vi "Arm Control.vi"(8 "error in (no error)":errorcluster) -> ()   [LabVIEW 2013]
uses:
  Robot Global Data.vi
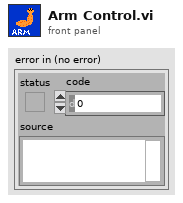
[diagram p1: front panel]
types:
  T1 = typedef "WPI_MotorControlDeviceRef.ctl" = cluster{"DeviceStatus":errorcluster, "Type":enum16{"PWM", "CAN"}, "PWM":cluster{"Digital Module":T2, "PWM Channel":T3, "DeadBand":T4}, "CAN":cluster{"Device Number":u8, "Control Mode":T5, "Semaphore":T6, "Max Vout":dbl}, "Invert":bool, "TransformRef":T7, "InvTransformRef":T7}
  T2 = typedef "FPGA_TypedefDigitalModule.ctl" = enum16{"Digital Module 1", "Digital Module 2"}
  T3 = typedef "FPGA_DIOPWMChannel.ctl" = enum8{"PWM 1", "PWM 2", "PWM 3", "PWM 4", "PWM 5", "PWM 6", "PWM 7", "PWM 8", "PWM 9", "PWM 10", "Invalid"}
  T4 = typedef "WPI_PWMDeadband.ctl" = cluster{"Name":string, "maxPositivePwm":i32, "minPositivePwm":i32, "centerPwm":i32, "maxNegativePwm":i32, "minNegativePwm":i32, "angularRange":u16}
  T5 = typedef "WPI_CANJaguar_ControlMode.ctl" = enum8{"Percent VBus", "Current", "Speed", "Position", "Voltage"}
  T6 = typedef "Semaphore RefNum" = refnum<k1>
  T7 = typedef "WPI_PWMTransform_ConPane.ctl" = refnum<vi>
  T8 = typedef "User Commands typedef.ctl" = cluster{"Arm Command":T9, "Shooter Commands":T11, "Drive Commands":T12}
  T9 = typedef "Arm control typedef.ctl" = cluster{"Arm up/dwn":dbl, "Arm Capture":bool, "Arm Pass":bool, "Arm Positions":T10, "Arm Manual Override":bool}
  T10 = typedef "Arm Postions Enum Typedef.ctl" = enum16{"Arm Pick-up", "Arm Shoot", "Arm Truss", "Manual"}
  T11 = typedef "Shooter Commands Typedef.ctl" = cluster{"Shooter Fire":bool, "Shooter Draw":bool}
  T12 = typedef "Drive Commands Typedef.ctl" = cluster{"Drive L/R":dbl, "Drive Fwd/Rev":dbl}
  T13 = typedef "Robot Info Typedef.ctl" = cluster{"Arm Info":T14, "Shooter Info":T15}
  T14 = typedef "Arm Info Typedef.ctl" = cluster{"Current Arm Position":dbl, "Arm Bottom Limit Switch":bool, "Arm Top Limit Switch":bool}
  T15 = typedef "Shooter Info Typedef.ctl" = cluster{"Shooter At Full":bool}
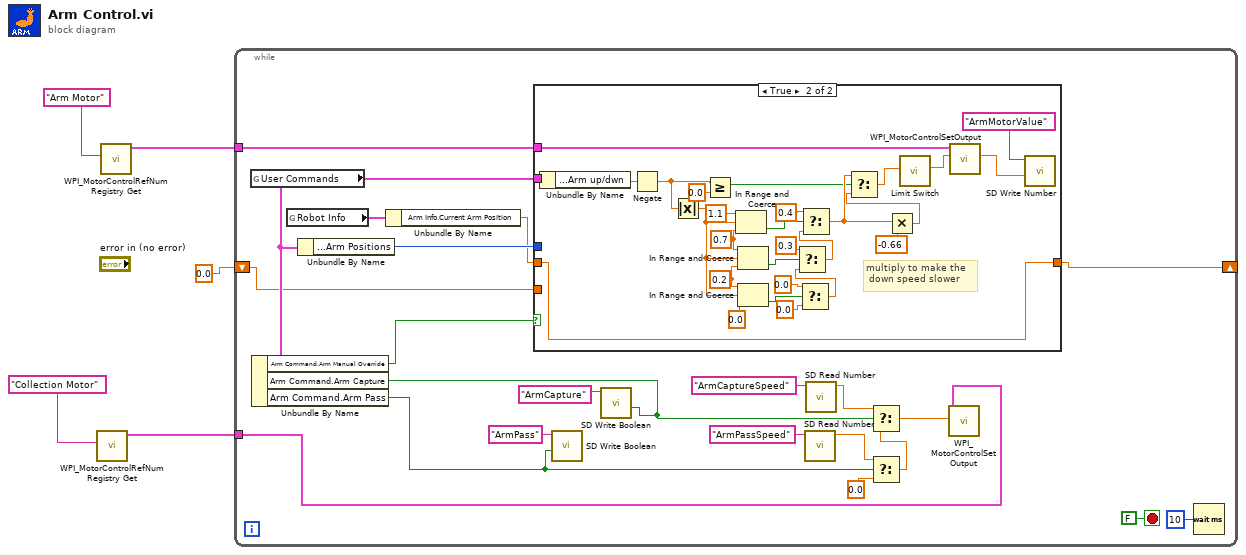
[diagram p0: block diagram]
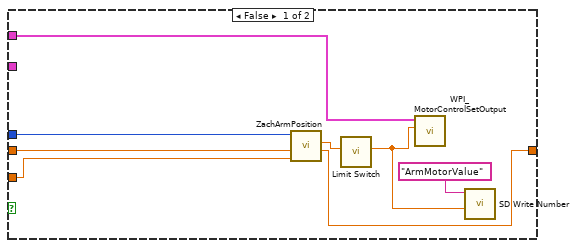
[diagram p2: hidden frame]
diagram:
  n1 = call <vilib>:"WPI_MotorControlRefNum Registry Get.vi"("refnum name"="Collection Motor") -> ("MotorControlDevRef"=w2:T1)  [unwired: 9 in, 1 out]
  n2 = call <vilib>:"WPI_MotorControlRefNum Registry Get.vi"("refnum name"="Arm Motor") -> ("MotorControlDevRef"=w4:T1)  [unwired: 9 in, 1 out]
  n3 = while {
    tunnel: w4 -> [w27]
    tunnel: w2 -> [w13]
    shift-right: [w7] -> _
    shift-left: 0.0 -> [w6]
    stop <- FALSE stop-if-true
    n4 = global read "Robot Global Data.vi" "User Commands"() -> (w12:T8)
    n5 = Unbundle By Name(w12) -> ("Arm Command.Arm Manual Override"=w10:bool, "Arm Command.Arm Capture"=w17:bool, "Arm Command.Arm Pass"=w16:bool)
    n6 = global read "Robot Global Data.vi" "Robot Info"() -> (w9:T13)
    n7 = Unbundle By Name(w12) -> ("Arm Command.Arm Positions"=w11:T10)
    n8 = Unbundle By Name(w9) -> ("Arm Info.Current Arm Position"=w8:dbl)
    n9 = case shown="True" w10 {
      tunnel: w27 -> [w35 w63]
      tunnel: w11 -> [w31 _]
      tunnel: w12 -> [_ w37]
      tunnel: w8 -> [w30 w36]
      tunnel: [w28 w36] -> w7
      tunnel: w6 -> [w29 _]
      frame False {
        n10 = call "ZachArmPosition.vi"("Manual Position"=w29, "Arm Position"=w30, "User Arm Position"=w31) -> ("Target Position"=w28:dbl, "Motor Speed"=w34:dbl)  [unwired: 7 in]
        n11 = call "Limit Switch.vi"("Input"=w34) -> ("Output"=w33:dbl)  [unwired: 10 in]
        n12 = call <vilib>:"WPI_MotorControlSetOutput.vi"("Output"=w33, "MotorControlDevRef"=w35) -> ()  [unwired: 7 in, 3 out]
        n13 = call <vilib>:"SD Write Number.vi"("Numeric"=w33, "Name"="ArmMotorValue") -> ()  [unwired: 8 in, 2 out]
      }
      frame True {
        w57 = 0.7 ("upper limit")
        w58 = 0.2 ("upper limit")
        # "multiply to make the\n down speed slower"
        n14 = Unbundle By Name(w37) -> ("Arm Command.Arm up/dwn"=w38:dbl)
        n15 = Negate(x=w38) -> (-x=w39:dbl)
        n16 = Absolute Value(x=w39) -> (abs(x)=w55:dbl)
        n17 = Greater Or Equal?(x=w39, y=0.0) -> (x >= y?=w40:bool)
        n18 = In Range and Coerce(upper limit=1.1, x=w55, lower limit=w57) -> (In Range?=w44:bool)  [unwired: 1 out]
        n19 = In Range and Coerce(upper limit=w57, x=w55, lower limit=w58) -> (In Range?=w50:bool)  [unwired: 1 out]
        n20 = In Range and Coerce(upper limit=w58, x=w55, lower limit=0.0) -> (In Range?=w49:bool)  [unwired: 1 out]
        n21 = Select(t=0.0, s=w49, f=0.0) -> (s? t:f=w51:dbl)
        n22 = Select(t=0.3, s=w50, f=w51) -> (s? t:f=w52:dbl)
        n23 = Select(t=0.4, s=w44, f=w52) -> (s? t:f=w41:dbl)
        n24 = Multiply(x=w41, y=-0.66) -> (x*y=w42:dbl)
        n25 = Select(t=w41, s=w40, f=w42) -> (s? t:f=w53:dbl)
        n26 = call "Limit Switch.vi"("Input"=w53) -> ("Output"=w60:dbl)  [unwired: 10 in]
        n27 = call <vilib>:"WPI_MotorControlSetOutput.vi"("Output"=w60, "MotorControlDevRef"=w63) -> ("Motor Output"=w62:dbl)  [unwired: 7 in, 2 out]
        n28 = call <vilib>:"SD Write Number.vi"("Numeric"=w62, "Name"="ArmMotorValue") -> ()  [unwired: 8 in, 2 out]
      }
    }
    n29 = call <vilib>:"SD Write Boolean.vi"("Boolean"=w16, "Name"="ArmPass") -> ()  [unwired: 8 in, 2 out]
    n30 = call <vilib>:"SD Write Boolean.vi"("Boolean"=w17, "Name"="ArmCapture") -> ()  [unwired: 8 in, 2 out]
    n31 = call <vilib>:"SD Read Number.vi"("Name"="ArmPassSpeed") -> ("Numeric"=w23:dbl)  [unwired: 8 in, 2 out]
    n32 = call <vilib>:"SD Read Number.vi"("Name"="ArmCaptureSpeed") -> ("Numeric"=w24:dbl)  [unwired: 8 in, 2 out]
    n33 = Select(t=w23, s=w16, f=0.0) -> (s? t:f=w22:dbl)
    n34 = Select(t=w24, s=w17, f=w22) -> (s? t:f=w20:dbl)
    n35 = call <vilib>:"WPI_MotorControlSetOutput.vi"("Output"=w20, "MotorControlDevRef"=w13) -> ()  [unwired: 7 in, 3 out]
    n36 = Wait (ms)(milliseconds to wait=u32 10) -> ()  [unwired: 1 out]
  }
